vi "Queue References FGV.vi"(8 "error in":errorcluster, 11 "function":enum16{"obtain", "get", "release"}(ring)) -> (0 "error out":errorcluster, 3 "module queues":T1)   [LabVIEW 2017, in "myPAM.lvlib"]
uses:
  myPAM.lvlib
  Private TypeDefs/Module Queues.ctl
  Private TypeDefs/Message Queue Element.ctl
  Global TypeDefs/Registered Modules.ctl
  Public TypeDefs/Messages.ctl
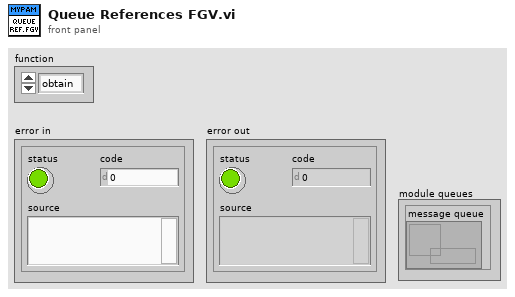
[diagram p1: front panel]
types:
  T1 = typedef "myPAM.lvlib/Module Queues.ctl" = cluster{"message queue":refnum<queue>}
  T2 = typedef "myPAM.lvlib/Message Queue Element.ctl" = cluster{"source":T3, "message":T4, "data":variant}
  T3 = typedef "Registered Modules.ctl" = enum16{"Controller", "DAQ", "Error Handler", "Game", "myPAM", "WinHost", "Logger"}
  T4 = typedef "myPAM.lvlib/Messages.ctl" = enum16{"calibrate encoders", "enable motors", "disable motors", "operate", "shutdown"}
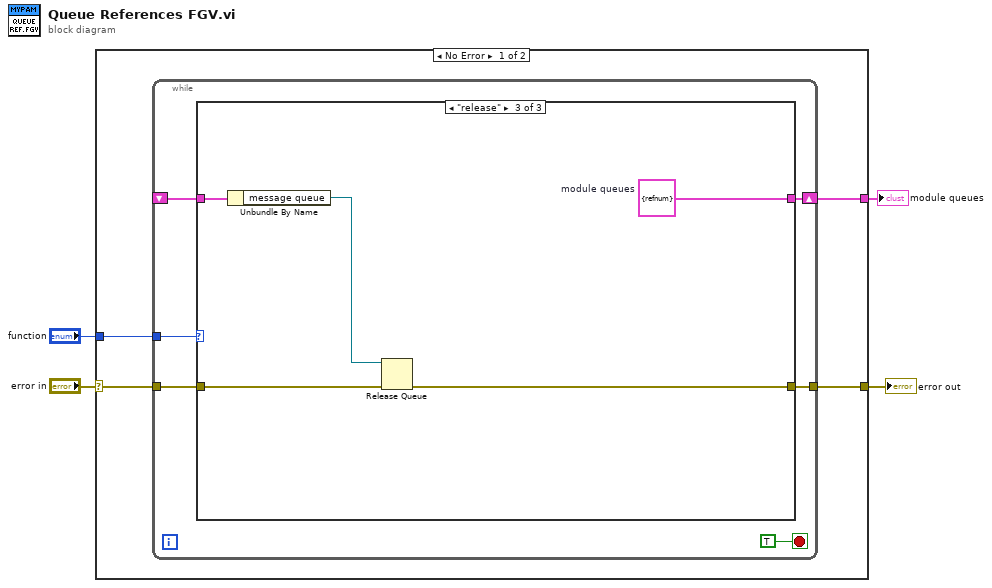
[diagram p0: block diagram]
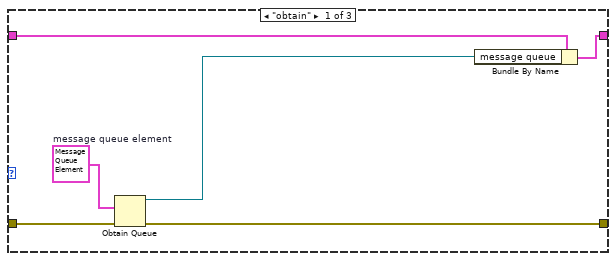
[diagram p2: hidden frame]
diagram:
  n1 = case shown="No Error" "error in" {
    selector: "error in" -> [w8 w28]
    tunnel: [w7 w28] -> w3
    tunnel: "function" -> [w6 _]
    tunnel: [w5 _] -> w1
    frame No Error {
      n2 = while {
        tunnel: w8 -> [w13]
        tunnel: [w12] -> w7
        tunnel: w6 -> [w11]
        shift-right: [w10] -> w5
        shift-left: _ -> [w9]
        stop <- TRUE stop-if-true
        n3 = case shown="\"release\"" w11 {
          tunnel: w13 -> [w20 w22 w27]
          tunnel: [w15 w22 w23] -> w12
          tunnel: [w16 w21 w24] -> w10
          tunnel: w9 -> [w18 w21 w26]
          frame "obtain" {
            w19 = T2 {"source"=enum."Controller", "message"=enum."calibrate encoders", "data"=variant}  # message queue element
            n4 = Obtain Queue(element data type=w19, error in (no error)=w20) -> (queue out=w17:refnum<queue>, error out=w15:errorcluster)  [unwired: 3 in, 1 out]
            n5 = Bundle By Name(cluster=w18, "message queue"=w17) -> (w16:T1)
          }
          frame "get", Default {
          }
          frame "release" {
            w24 = T1 {"message queue"=refnum}  # module queues
            n6 = Unbundle By Name(w26) -> ("message queue"=w25:refnum<queue>)
            n7 = Release Queue(queue=w25, error in (no error)=w27) -> (error out=w23:errorcluster)  [unwired: 1 in, 2 out]
          }
        }
      }
    }
    frame Error {
    }
  }
  "error out" <- w3
  "module queues" <- w1
